vi "meth.PullReturns.vi"(0 "class.GLue in":refnum<class "class.GLue.lvclass">, 2 "ScriptReturn":bool, 11 "error in":errorcluster) -> (4 "class.GLue out":refnum<class "class.GLue.lvclass">, 15 "error out":errorcluster)   [LabVIEW 2014, in "GLue.lvlib" / "class.GLue.lvclass"]
uses:
  class.GLue.lvclass
  class.GLue.lvclass/class.GLue.ctl
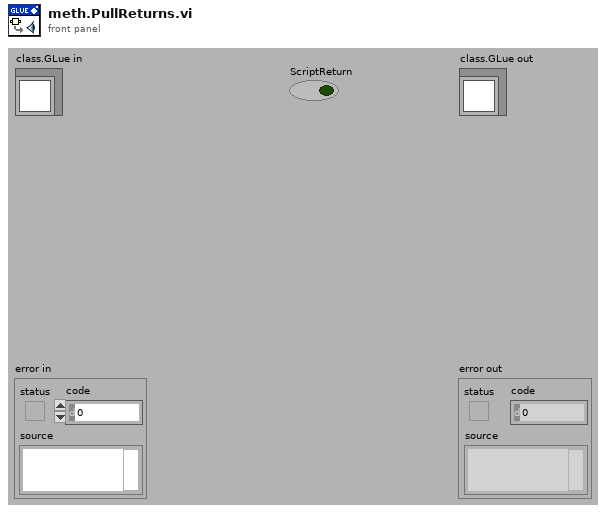
[diagram p1: front panel]
types:
  T1 = typedef "GLue.lvlib/class.GLue.lvclass/typedef.Types.ctl" = enum16{"Nil", "Bool", "LightUserData", "Number", "String", "Table", "Function", "UserData", "Thread"}
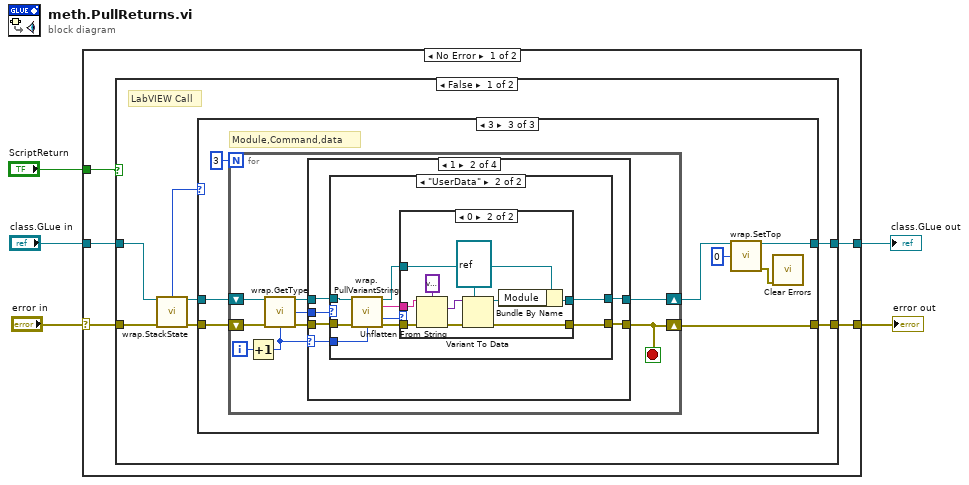
[diagram p0: block diagram]
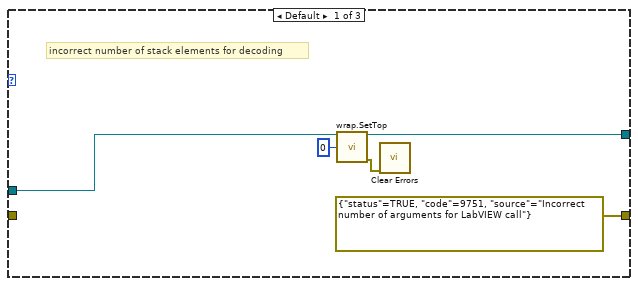
[diagram p2: hidden frame]
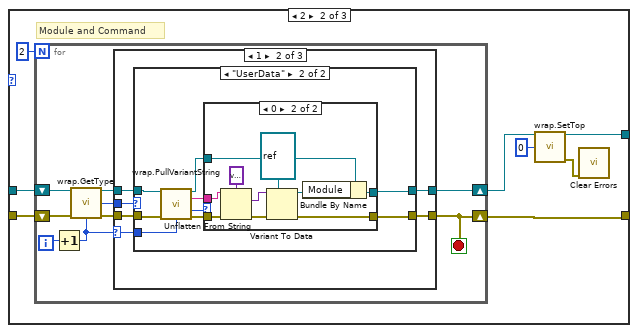
[diagram p3: hidden frame]
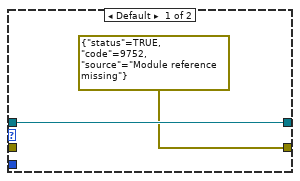
[diagram p5: hidden frame]
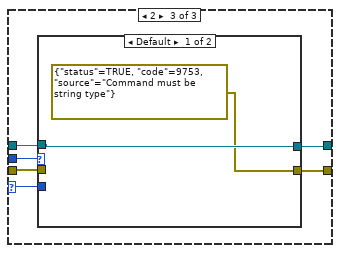
[diagram p7: hidden frame]
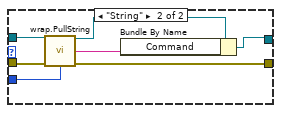
[diagram p8: hidden frame]
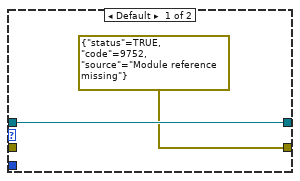
[diagram p10: hidden frame]
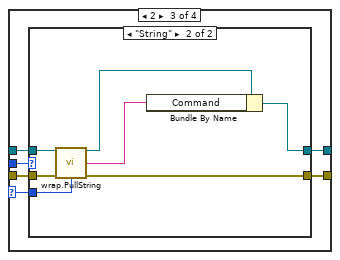
[diagram p12: hidden frame]
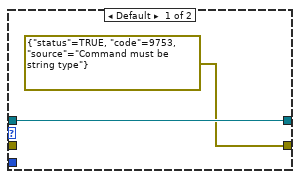
[diagram p13: hidden frame]
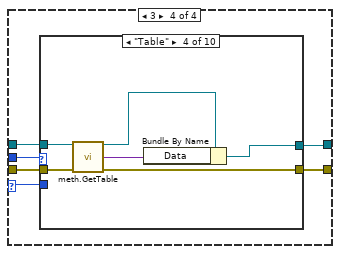
[diagram p14: hidden frame]
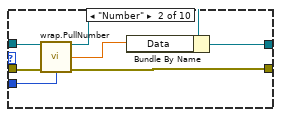
[diagram p16: hidden frame]
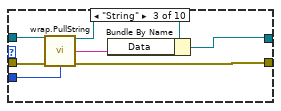
[diagram p17: hidden frame]
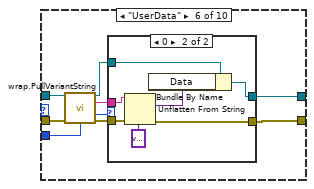
[diagram p19: hidden frame]
diagram:
  n1 = case shown="No Error" "error in" {
    selector: "error in" -> [w9 w362]
    tunnel: [w8 w362] -> w4
    tunnel: [w7 w361] -> w2
    tunnel: "class.GLue in" -> [w10 w361]
    tunnel: "ScriptReturn" -> [w6 _]
    frame No Error {
      n2 = case shown="False" w6 {
        tunnel: w10 -> [w17 w210]
        tunnel: w9 -> [w16 w213]
        tunnel: [w15 w211] -> w8
        tunnel: [w14 w212] -> w7
        frame False {
          # "LabVIEW Call"
          n3 = call "wrap.StackState.vi"("class.GLue in"=w17, "error in (no error)"=w16) -> ("class.GLue out"=w12:refnum<class "class.GLue.lvclass">, "Size"=w11:i32, "error out"=w13:errorcluster)  [unwired: 10 in, 1 out]
          n4 = case shown="3" w11 {
            tunnel: w13 -> [_ w30 w93]
            tunnel: w12 -> [w20 w29 w92]
            tunnel: [errorcluster {"status"=TRUE, "code"=9751, "source"="Incorrect number of arguments for LabVIEW call"} ("error out") w24 w87] -> w15
            tunnel: [w19 w27 w90] -> w14
            frame Default {
              # "incorrect number of stack elements for decoding"
              n5 = call "wrap.SetTop.vi"("class.GLue in"=w20, "Index"=0) -> ("class.GLue out"=w19:refnum<class "class.GLue.lvclass">, "error out"=w22:errorcluster)  [unwired: 12 in]
              n6 = call <vilib>:"Clear Errors.vi"("error in (no error)"=w22) -> ()  [unwired: 5 in, 2 out]
            }
            frame 2 {
              # "Module and Command"
              n7 = for {
                N: 2 -> [_]
                shift-right: [w34] -> w26
                shift-left: w29 -> [w38]
                shift-right: [w33] -> w24
                shift-left: w30 -> [w39]
                i -> [w32]
                stop <- w33 stop-if-true
                n8 = Increment(x=w32) -> (x+1=w31:i32)
                n9 = call "wrap.GetType.vi"("class.GLue in"=w38, "error in (no error)"=w39, "Index"=w31) -> ("class.GLue out"=w35:refnum<class "class.GLue.lvclass">, "Type"=w37:T1, "error out"=w36:errorcluster)  [unwired: 10 in]
                n10 = case shown="1" w31 {
                  selector: w31 -> [_ w42 w73]
                  tunnel: w37 -> [_ w47 w74]
                  tunnel: w36 -> [w40 w46 w75]
                  tunnel: w35 -> [w41 w45 w76]
                  tunnel: [w41 w44 w72] -> w34
                  tunnel: [w40 w43 w71] -> w33
                  frame Default {
                  }
                  frame 1 {
                    n11 = case shown="\"UserData\"" w47 {
                      tunnel: w46 -> [_ w53]
                      tunnel: w45 -> [w49 w54]
                      tunnel: w42 -> [_ w50]
                      tunnel: [errorcluster {"status"=TRUE, "code"=9752, "source"="Module reference missing"} ("error out") w52] -> w43
                      tunnel: [w49 w51] -> w44
                      frame Default {
                      }
                      frame "UserData" {
                        n12 = call "wrap.PullVariantString.vi"("class.GLue in"=w54, "error in (no error)"=w53, "Index"=w50) -> ("class.GLue out"=w58:refnum<class "class.GLue.lvclass">, "VarString"=w57:string, "Return"=w55:i32, "error out"=w56:errorcluster)  [unwired: 9 in]
                        n13 = case shown="0" w55 {
                          tunnel: w56 -> [w60 w70]
                          tunnel: w57 -> [_ w69]
                          tunnel: w58 -> [w59 w67]
                          tunnel: [w59 w66] -> w51
                          tunnel: [w60 w62] -> w52
                          frame Default {
                          }
                          frame 0 {
                            n14 = Unflatten From String(type=variant ("Cluster"), binary string=w69, error in (no error)=w70) -> (value=w64:variant, error out=w65:errorcluster)  [unwired: 2 in, 1 out]
                            n15 = Variant To Data(error in=w65, type=refnum<vi> refnum ("Module"), Variant=w64) -> (data=w63:refnum<vi>, error out=w62:errorcluster)
                            n16 = Bundle By Name(cluster=w67, "Module"=w63) -> (w66:refnum<class "class.GLue.lvclass">)
                          }
                        }
                      }
                    }
                  }
                  frame 2 {
                    n17 = case shown="Default" w74 {
                      tunnel: w75 -> [_ w85]
                      tunnel: w76 -> [w78 w84]
                      tunnel: w73 -> [_ w79]
                      tunnel: [errorcluster {"status"=TRUE, "code"=9753, "source"="Command must be string type"} ("error out") w80] -> w71
                      tunnel: [w78 w81] -> w72
                      frame Default {
                      }
                      frame "String" {
                        n18 = call "wrap.PullString.vi"("class.GLue in"=w84, "error in (no error)"=w85, "Index"=w79) -> ("class.GLue out"=w83:refnum<class "class.GLue.lvclass">, "String"=w82:string, "error out"=w80:errorcluster)  [unwired: 10 in]
                        n19 = Bundle By Name(cluster=w83, "Command"=w82) -> (w81:refnum<class "class.GLue.lvclass">)
                      }
                    }
                  }
                }
              }
              n20 = call "wrap.SetTop.vi"("class.GLue in"=w26, "Index"=0) -> ("class.GLue out"=w27:refnum<class "class.GLue.lvclass">, "error out"=w23:errorcluster)  [unwired: 12 in]
              n21 = call <vilib>:"Clear Errors.vi"("error in (no error)"=w23) -> ()  [unwired: 5 in, 2 out]
            }
            frame 3 {
              # "Module,Command,data"
              n22 = for {
                N: 3 -> [_]
                shift-right: [w97] -> w89
                shift-left: w92 -> [w101]
                shift-right: [w96] -> w87
                shift-left: w93 -> [w102]
                i -> [w95]
                stop <- w96 stop-if-true
                n23 = Increment(x=w95) -> (x+1=w94:i32)
                n24 = call "wrap.GetType.vi"("class.GLue in"=w101, "error in (no error)"=w102, "Index"=w94) -> ("class.GLue out"=w98:refnum<class "class.GLue.lvclass">, "Type"=w100:T1, "error out"=w99:errorcluster)  [unwired: 10 in]
                n25 = case shown="1" w94 {
                  selector: w94 -> [_ w105 w134 w151]
                  tunnel: w100 -> [_ w106 w139 w153]
                  tunnel: w99 -> [w103 w109 w138 w152]
                  tunnel: w98 -> [w104 w110 w137 w154]
                  tunnel: [w104 w108 w136 w150] -> w97
                  tunnel: [w103 w107 w135 w149] -> w96
                  frame Default {
                  }
                  frame 1 {
                    n26 = case shown="\"UserData\"" w106 {
                      tunnel: w109 -> [_ w116]
                      tunnel: w110 -> [w112 w117]
                      tunnel: [errorcluster {"status"=TRUE, "code"=9752, "source"="Module reference missing"} ("error out") w115] -> w107
                      tunnel: [w112 w114] -> w108
                      tunnel: w105 -> [_ w113]
                      frame Default {
                      }
                      frame "UserData" {
                        n27 = call "wrap.PullVariantString.vi"("class.GLue in"=w117, "error in (no error)"=w116, "Index"=w113) -> ("class.GLue out"=w121:refnum<class "class.GLue.lvclass">, "VarString"=w120:string, "Return"=w118:i32, "error out"=w119:errorcluster)  [unwired: 9 in]
                        n28 = case shown="0" w118 {
                          tunnel: w119 -> [w123 w133]
                          tunnel: w120 -> [_ w132]
                          tunnel: w121 -> [w122 w130]
                          tunnel: [w122 w129] -> w114
                          tunnel: [w123 w125] -> w115
                          frame Default {
                          }
                          frame 0 {
                            n29 = Unflatten From String(type=variant ("Cluster"), binary string=w132, error in (no error)=w133) -> (value=w127:variant, error out=w128:errorcluster)  [unwired: 2 in, 1 out]
                            n30 = Variant To Data(error in=w128, type=refnum<vi> refnum ("Module"), Variant=w127) -> (data=w126:refnum<vi>, error out=w125:errorcluster)
                            n31 = Bundle By Name(cluster=w130, "Module"=w126) -> (w129:refnum<class "class.GLue.lvclass">)
                          }
                        }
                      }
                    }
                  }
                  frame 2 {
                    n32 = case shown="\"String\"" w139 {
                      tunnel: w138 -> [_ w148]
                      tunnel: w137 -> [w141 w146]
                      tunnel: w134 -> [_ w147]
                      tunnel: [errorcluster {"status"=TRUE, "code"=9753, "source"="Command must be string type"} ("error out") w144] -> w135
                      tunnel: [w141 w143] -> w136
                      frame Default {
                      }
                      frame "String" {
                        n33 = call "wrap.PullString.vi"("class.GLue in"=w146, "error in (no error)"=w148, "Index"=w147) -> ("class.GLue out"=w145:refnum<class "class.GLue.lvclass">, "String"=w142:string, "error out"=w144:errorcluster)  [unwired: 10 in]
                        n34 = Bundle By Name(cluster=w145, "Command"=w142) -> (w143:refnum<class "class.GLue.lvclass">)
                      }
                    }
                  }
                  frame 3 {
                    n35 = case shown="\"Table\"" w153 {
                      tunnel: w152 -> [w156 w163 w170 w176 w177 w187 w198 w200 w207 w209]
                      tunnel: w154 -> [w155 w161 w169 w175 w178 w186 w197 w199 w206 w208]
                      tunnel: w151 -> [_ w162 w164 _ _ w179 _ _ w205 _]
                      tunnel: [w156 w158 w165 w171 w177 w180 w198 w200 w201 w209] -> w149
                      tunnel: [w155 w157 w166 w173 w178 w181 w197 w199 w202 w208] -> w150
                      frame Default {
                      }
                      frame "Number" {
                        n36 = call "wrap.PullNumber.vi"("class.GLue in"=w161, "error in (no error)"=w163, "Index"=w162) -> ("class.GLue out"=w160:refnum<class "class.GLue.lvclass">, "Number"=w159:dbl, "error out"=w158:errorcluster)  [unwired: 10 in]
                        n37 = Bundle By Name(cluster=w160, "Data"=w159) -> (w157:refnum<class "class.GLue.lvclass">)
                      }
                      frame "String" {
                        n38 = call "wrap.PullString.vi"("class.GLue in"=w169, "error in (no error)"=w170, "Index"=w164) -> ("class.GLue out"=w168:refnum<class "class.GLue.lvclass">, "String"=w167:string, "error out"=w165:errorcluster)  [unwired: 10 in]
                        n39 = Bundle By Name(cluster=w168, "Data"=w167) -> (w166:refnum<class "class.GLue.lvclass">)
                      }
                      frame "Table" {
                        n40 = call "meth.GetTable.vi"("class.GLue in"=w175, "error in (no error)"=w176) -> ("class.GLue out"=w174:refnum<class "class.GLue.lvclass">, "Table"=w172:variant, "error out"=w171:errorcluster)  [unwired: 11 in]
                        n41 = Bundle By Name(cluster=w174, "Data"=w172) -> (w173:refnum<class "class.GLue.lvclass">)
                      }
                      frame "Function" {
                      }
                      frame "UserData" {
                        n42 = call "wrap.PullVariantString.vi"("class.GLue in"=w186, "error in (no error)"=w187, "Index"=w179) -> ("class.GLue out"=w182:refnum<class "class.GLue.lvclass">, "VarString"=w183:string, "Return"=w185:i32, "error out"=w184:errorcluster)  [unwired: 9 in]
                        n43 = case shown="0" w185 {
                          tunnel: w184 -> [w189 w196]
                          tunnel: w183 -> [_ w195]
                          tunnel: w182 -> [w188 w193]
                          tunnel: [w188 w191] -> w181
                          tunnel: [w189 w190] -> w180
                          frame Default {
                          }
                          frame 0 {
                            n44 = Unflatten From String(type=variant ("Cluster"), binary string=w195, error in (no error)=w196) -> (value=w192:variant, error out=w190:errorcluster)  [unwired: 2 in, 1 out]
                            n45 = Bundle By Name(cluster=w193, "Data"=w192) -> (w191:refnum<class "class.GLue.lvclass">)
                          }
                        }
                      }
                      frame "Thread" {
                      }
                      frame "LightUserData" {
                      }
                      frame "Bool" {
                        n46 = call "wrap.PullBool.vi"("class.GLue in"=w206, "error in (no error)"=w207, "Index"=w205) -> ("class.GLue out"=w204:refnum<class "class.GLue.lvclass">, "Boolean"=w203:bool, "error out"=w201:errorcluster)  [unwired: 10 in]
                        n47 = Bundle By Name(cluster=w204, "Data"=w203) -> (w202:refnum<class "class.GLue.lvclass">)
                      }
                      frame "Nil" {
                      }
                    }
                  }
                }
              }
              n48 = call "wrap.SetTop.vi"("class.GLue in"=w89, "Index"=0) -> ("class.GLue out"=w90:refnum<class "class.GLue.lvclass">, "error out"=w86:errorcluster)  [unwired: 12 in]
              n49 = call <vilib>:"Clear Errors.vi"("error in (no error)"=w86) -> ()  [unwired: 5 in, 2 out]
            }
          }
        }
        frame True {
          n50 = call "wrap.StackState.vi"("class.GLue in"=w210, "error in (no error)"=w213) -> ("class.GLue out"=w215:refnum<class "class.GLue.lvclass">, "Size"=w214:i32, "error out"=w216:errorcluster)  [unwired: 10 in, 1 out]
          n51 = case shown="2" w214 {
            tunnel: w216 -> [w217 w222 w239 w305]
            tunnel: w215 -> [w218 w225 w238 w295]
            tunnel: [w217 w222 w233 w300] -> w211
            tunnel: [w219 w226 w236 w303] -> w212
            frame Default {
              # "incorrect number of stack elements for decoding"
              n52 = call "wrap.SetTop.vi"("class.GLue in"=w218, "Index"=0) -> ("class.GLue out"=w219:refnum<class "class.GLue.lvclass">, "error out"=w221:errorcluster)  [unwired: 12 in]
              n53 = call <vilib>:"Clear Errors.vi"("error in (no error)"=w221) -> ()  [unwired: 5 in, 2 out]
            }
            frame 0 {
              # "Basic returns, with no 'Data' field"
              n54 = Bundle By Name(cluster=w225, "Data"=variant ("LVCall.Data")) -> (w224:refnum<class "class.GLue.lvclass">)
              n55 = call "wrap.SetTop.vi"("class.GLue in"=w224, "Index"=0) -> ("class.GLue out"=w226:refnum<class "class.GLue.lvclass">, "error out"=w228:errorcluster)  [unwired: 12 in]
              n56 = call <vilib>:"Clear Errors.vi"("error in (no error)"=w228) -> ()  [unwired: 5 in, 2 out]
            }
            frame 1 {
              w229 = -1 ("Index")
              # "Normal return, with 'Data'"
              n57 = call "wrap.GetType.vi"("class.GLue in"=w238, "error in (no error)"=w239, "Index"=w229) -> ("class.GLue out"=w230:refnum<class "class.GLue.lvclass">, "Type"=w232:T1, "error out"=w231:errorcluster)  [unwired: 10 in]
              n58 = case shown="\"Table\"" w232 {
                tunnel: w231 -> [w241 w248 w255 w256 w262 w272 w283 w285 w292 w294]
                tunnel: w230 -> [w240 w246 w254 w257 w263 w271 w282 w284 w291 w293]
                tunnel: w229 -> [_ w247 w249 _ _ w264 _ _ w290 _]
                tunnel: [w241 w243 w250 w260 w262 w265 w283 w285 w286 w294] -> w233
                tunnel: [w240 w242 w251 w258 w263 w266 w282 w284 w287 w293] -> w237
                frame Default {
                }
                frame "Number" {
                  n59 = call "wrap.PullNumber.vi"("class.GLue in"=w246, "error in (no error)"=w248, "Index"=w247) -> ("class.GLue out"=w245:refnum<class "class.GLue.lvclass">, "Number"=w244:dbl, "error out"=w243:errorcluster)  [unwired: 10 in]
                  n60 = Bundle By Name(cluster=w245, "Data"=w244) -> (w242:refnum<class "class.GLue.lvclass">)
                }
                frame "String" {
                  n61 = call "wrap.PullString.vi"("class.GLue in"=w254, "error in (no error)"=w255, "Index"=w249) -> ("class.GLue out"=w253:refnum<class "class.GLue.lvclass">, "String"=w252:string, "error out"=w250:errorcluster)  [unwired: 10 in]
                  n62 = Bundle By Name(cluster=w253, "Data"=w252) -> (w251:refnum<class "class.GLue.lvclass">)
                }
                frame "Table" {
                  n63 = call "meth.GetTable.vi"("class.GLue in"=w257, "error in (no error)"=w256) -> ("class.GLue out"=w259:refnum<class "class.GLue.lvclass">, "Table"=w261:variant, "error out"=w260:errorcluster)  [unwired: 11 in]
                  n64 = Bundle By Name(cluster=w259, "Data"=w261) -> (w258:refnum<class "class.GLue.lvclass">)
                }
                frame "Function" {
                }
                frame "UserData" {
                  n65 = call "wrap.PullVariantString.vi"("class.GLue in"=w271, "error in (no error)"=w272, "Index"=w264) -> ("class.GLue out"=w267:refnum<class "class.GLue.lvclass">, "VarString"=w268:string, "Return"=w270:i32, "error out"=w269:errorcluster)  [unwired: 9 in]
                  n66 = case shown="0" w270 {
                    tunnel: w269 -> [w274 w281]
                    tunnel: w268 -> [_ w280]
                    tunnel: w267 -> [w273 w278]
                    tunnel: [w273 w276] -> w266
                    tunnel: [w274 w275] -> w265
                    frame Default {
                    }
                    frame 0 {
                      n67 = Unflatten From String(type=variant ("Cluster"), binary string=w280, error in (no error)=w281) -> (value=w277:variant, error out=w275:errorcluster)  [unwired: 2 in, 1 out]
                      n68 = Bundle By Name(cluster=w278, "Data"=w277) -> (w276:refnum<class "class.GLue.lvclass">)
                    }
                  }
                }
                frame "Thread" {
                }
                frame "LightUserData" {
                }
                frame "Bool" {
                  n69 = call "wrap.PullBool.vi"("class.GLue in"=w291, "error in (no error)"=w292, "Index"=w290) -> ("class.GLue out"=w289:refnum<class "class.GLue.lvclass">, "Boolean"=w288:bool, "error out"=w286:errorcluster)  [unwired: 10 in]
                  n70 = Bundle By Name(cluster=w289, "Data"=w288) -> (w287:refnum<class "class.GLue.lvclass">)
                }
                frame "Nil" {
                }
              }
              n71 = call "wrap.SetTop.vi"("class.GLue in"=w237, "Index"=0) -> ("class.GLue out"=w236:refnum<class "class.GLue.lvclass">, "error out"=w235:errorcluster)  [unwired: 12 in]
              n72 = call <vilib>:"Clear Errors.vi"("error in (no error)"=w235) -> ()  [unwired: 5 in, 2 out]
            }
            frame 2 {
              w296 = -1 ("Index")
              # "return from pcalled function.. pcall still on stack - top most value is return"
              n73 = call "wrap.GetType.vi"("class.GLue in"=w295, "error in (no error)"=w305, "Index"=w296) -> ("class.GLue out"=w297:refnum<class "class.GLue.lvclass">, "Type"=w299:T1, "error out"=w298:errorcluster)  [unwired: 10 in]
              n74 = case shown="\"UserData\"" w299 {
                tunnel: w298 -> [w307 w314 w321 w322 w328 w338 w349 w351 w358 w360]
                tunnel: w297 -> [w306 w312 w320 w323 w329 w337 w348 w350 w357 w359]
                tunnel: w296 -> [_ w313 w315 _ _ w330 _ _ w356 _]
                tunnel: [w307 w309 w316 w326 w328 w331 w349 w351 w352 w360] -> w300
                tunnel: [w306 w308 w317 w324 w329 w332 w348 w350 w353 w359] -> w304
                frame Default {
                }
                frame "Number" {
                  n75 = call "wrap.PullNumber.vi"("class.GLue in"=w312, "error in (no error)"=w314, "Index"=w313) -> ("class.GLue out"=w311:refnum<class "class.GLue.lvclass">, "Number"=w310:dbl, "error out"=w309:errorcluster)  [unwired: 10 in]
                  n76 = Bundle By Name(cluster=w311, "Data"=w310) -> (w308:refnum<class "class.GLue.lvclass">)
                }
                frame "String" {
                  n77 = call "wrap.PullString.vi"("class.GLue in"=w320, "error in (no error)"=w321, "Index"=w315) -> ("class.GLue out"=w319:refnum<class "class.GLue.lvclass">, "String"=w318:string, "error out"=w316:errorcluster)  [unwired: 10 in]
                  n78 = Bundle By Name(cluster=w319, "Data"=w318) -> (w317:refnum<class "class.GLue.lvclass">)
                }
                frame "Table" {
                  n79 = call "meth.GetTable.vi"("class.GLue in"=w323, "error in (no error)"=w322) -> ("class.GLue out"=w325:refnum<class "class.GLue.lvclass">, "Table"=w327:variant, "error out"=w326:errorcluster)  [unwired: 11 in]
                  n80 = Bundle By Name(cluster=w325, "Data"=w327) -> (w324:refnum<class "class.GLue.lvclass">)
                }
                frame "Function" {
                }
                frame "UserData" {
                  n81 = call "wrap.PullVariantString.vi"("class.GLue in"=w337, "error in (no error)"=w338, "Index"=w330) -> ("class.GLue out"=w333:refnum<class "class.GLue.lvclass">, "VarString"=w334:string, "Return"=w336:i32, "error out"=w335:errorcluster)  [unwired: 9 in]
                  n82 = case shown="0" w336 {
                    tunnel: w335 -> [w340 w347]
                    tunnel: w334 -> [_ w346]
                    tunnel: w333 -> [w339 w344]
                    tunnel: [w339 w342] -> w332
                    tunnel: [w340 w341] -> w331
                    frame Default {
                    }
                    frame 0 {
                      n83 = Unflatten From String(type=variant ("Cluster"), binary string=w346, error in (no error)=w347) -> (value=w343:variant, error out=w341:errorcluster)  [unwired: 2 in, 1 out]
                      n84 = Bundle By Name(cluster=w344, "Data"=w343) -> (w342:refnum<class "class.GLue.lvclass">)
                    }
                  }
                }
                frame "Thread" {
                }
                frame "LightUserData" {
                }
                frame "Bool" {
                  n85 = call "wrap.PullBool.vi"("class.GLue in"=w357, "error in (no error)"=w358, "Index"=w356) -> ("class.GLue out"=w355:refnum<class "class.GLue.lvclass">, "Boolean"=w354:bool, "error out"=w352:errorcluster)  [unwired: 10 in]
                  n86 = Bundle By Name(cluster=w355, "Data"=w354) -> (w353:refnum<class "class.GLue.lvclass">)
                }
                frame "Nil" {
                }
              }
              n87 = call "wrap.SetTop.vi"("class.GLue in"=w304, "Index"=0) -> ("class.GLue out"=w303:refnum<class "class.GLue.lvclass">, "error out"=w302:errorcluster)  [unwired: 12 in]
              n88 = call <vilib>:"Clear Errors.vi"("error in (no error)"=w302) -> ()  [unwired: 5 in, 2 out]
            }
          }
        }
      }
    }
    frame Error {
    }
  }
  "error out" <- w4
  "class.GLue out" <- w2
